vi "TCP Server 全双工.vi"() -> ()   [LabVIEW 2015]
uses:
  <vilib>/measure/NI_MABase.lvlib
panel:
  in  "stop 2":bool
  in  "stop":bool
  out "receive from client":dbl[](graph)
  in  "port":u16
  out "send to client":waveform(dbl)(graph)
  in  "signal type":T1(ring)
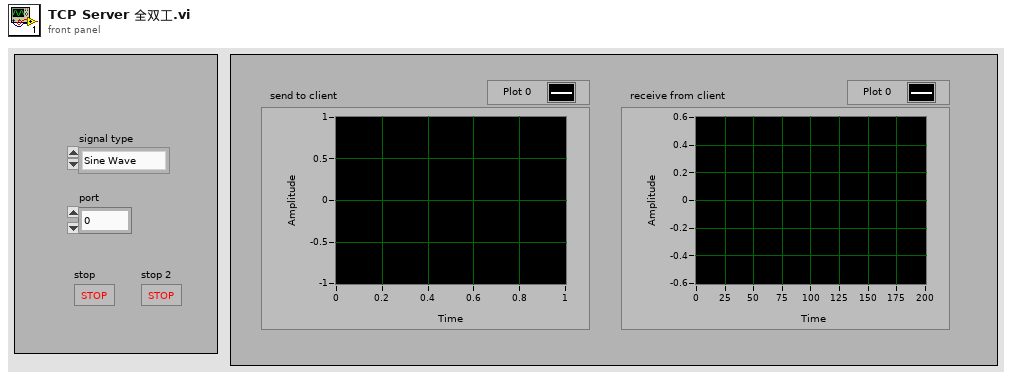
[diagram p1: front panel]
types:
  T1 = enum16{"Sine Wave", "Triangle Wave", "Square Wave", "Sawtooth Wave"}
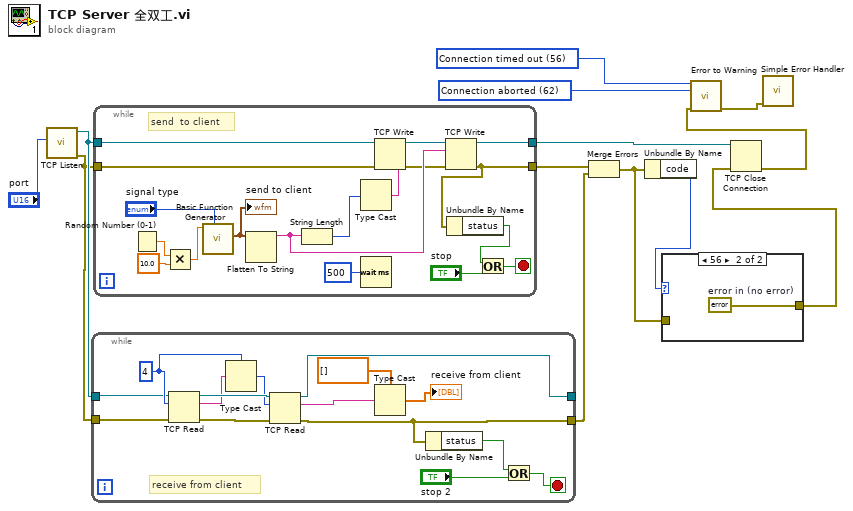
[diagram p0: block diagram]
diagram:
  w6 = 62 items=["No Error", "Argument Error", "Memory Full", "Out of Zone", "End of File", "File Already Open", "Generic File IO Error", "File Not Found", "File Permission Error", "Disk Full", "Duplicate Path", "Too Many Files Open", "Not Enabled", "Resource File Not Found", "Cannot Add Resource", "Resource Not Found", "Image Not Found", "Image Memory Error", "Pen Does Not Exist", "Config Bad Type", "Config Token Not Found", "Config Parse Error", "Config Memory Error", "Bad External Code Format", "Bad External Code Offset", "External Code Not Present", "Null Window", "Destroy Window Mixup", "Null Menu", "Print Aborted", "Bad Print Record", "Print Driver Error", "Windows Error During Print", "Memory Error During Print", "Print Dialog Error", "Generic Print Error", "Invalid Device Refnum", "Device Not Found", "Device Parameter Error", "Device Unit Error", "Can't Open Device", "Device Call Aborted", "Generic Error", "Cancelled By User", "Object ID Too Low", "Object ID Too High", "Object Not In Heap", "Unknown Heap", "Bad DefProc ID", "DefProc Not In Table", "Message Out Of Range", "Null Method", "Unknown Message", "Manager Call Not Supported", "Bad address", "Connection In progress", "Connection timed out", "Connection is already in progress", "Network attribute not supported", "Network error", "Address in use", "System out of memory", "Connection aborted", "Connection refused", "Connection is not connected", "Connection is already connected", "Connection closed", "Initialize error (interapplication manager)", "Bad occurrence", "Wait on unbound occurrence handler", "Occurrence queue overflow", "Bad path", "Semaphore not signaled", "Unrecognized type (interapplication manager)"] ("2nd Error to Convert")
  w7 = 56 items=["No Error", "Argument Error", "Memory Full", "Out of Zone", "End of File", "File Already Open", "Generic File IO Error", "File Not Found", "File Permission Error", "Disk Full", "Duplicate Path", "Too Many Files Open", "Not Enabled", "Resource File Not Found", "Cannot Add Resource", "Resource Not Found", "Image Not Found", "Image Memory Error", "Pen Does Not Exist", "Config Bad Type", "Config Token Not Found", "Config Parse Error", "Config Memory Error", "Bad External Code Format", "Bad External Code Offset", "External Code Not Present", "Null Window", "Destroy Window Mixup", "Null Menu", "Print Aborted", "Bad Print Record", "Print Driver Error", "Windows Error During Print", "Memory Error During Print", "Print Dialog Error", "Generic Print Error", "Invalid Device Refnum", "Device Not Found", "Device Parameter Error", "Device Unit Error", "Can't Open Device", "Device Call Aborted", "Generic Error", "Cancelled By User", "Object ID Too Low", "Object ID Too High", "Object Not In Heap", "Unknown Heap", "Bad DefProc ID", "DefProc Not In Table", "Message Out Of Range", "Null Method", "Unknown Message", "Manager Call Not Supported", "Bad address", "Connection In progress", "Connection timed out", "Connection is already in progress", "Network attribute not supported", "Network error", "Address in use", "System out of memory", "Connection aborted", "Connection refused", "Connection is not connected", "Connection is already connected", "Connection closed", "Initialize error (interapplication manager)", "Bad occurrence", "Wait on unbound occurrence handler", "Occurrence queue overflow", "Bad path", "Semaphore not signaled", "Unrecognized type (interapplication manager)"] ("1st Error to Convert")
  n1 = call <vilib>:"TCP Listen.vi"("port"="port") -> ("error out"=w5:errorcluster, "connection ID"=w10:refnum<k5>)  [unwired: 6 in, 3 out]
  n2 = while {
    tunnel: [w22] -> _
    tunnel: [w16] -> w12
    tunnel: w10 -> [w21]
    tunnel: w5 -> [w19]
    stop <- w20 stop-if-true
    w26 = 4
    # "receive from client"
    n3 = TCP Read(connection ID=w21, bytes to read=w26, error in (no error)=w19) -> (connection ID out=w28:refnum<k5>, data out=w25:string, error out=w27:errorcluster)  [unwired: 2 in]
    n4 = Type Cast(type=w26, x=w25) -> (*(type *) &x=w24:i32)
    n5 = TCP Read(connection ID=w28, bytes to read=w24, error in (no error)=w27) -> (connection ID out=w22:refnum<k5>, data out=w23:string, error out=w16:errorcluster)  [unwired: 2 in]
    n6 = Type Cast(type=dbl[] [], x=w23) -> (*(type *) &x=→"receive from client":dbl[])
    n7 = Unbundle By Name(w16) -> ("status"=w18:bool)
    n8 = Or(x=w18, y="stop 2") -> (x .or. y?=w20:bool)
  }
  n9 = while {
    tunnel: [w36] -> w11
    tunnel: w10 -> [w35]
    tunnel: w5 -> [w34]
    tunnel: [w32] -> w9
    stop <- w33 stop-if-true
    # "send  to client"
    n10 = Random Number (0-1)() -> (number: 0 to 1=w45:dbl)
    n11 = Multiply(x=w45, y=10.0) -> (x*y=w43:dbl)
    n12 = call <vilib>:"Basic Function Generator.vi"("signal type"="signal type", "frequency"=w43) -> ("signal out"=w41:waveform(dbl))  [unwired: 7 in, 2 out]
    "send to client" <- w41
    n13 = Flatten To String(anything=w41) -> (data string=w39:string)  [unwired: 3 in, 2 out]
    n14 = String Length(string=w39) -> (length=w42:i32)
    n15 = Type Cast(x=w42) -> (*(type *) &x=w40:string)  [unwired: 1 in]
    n16 = Wait (ms)(milliseconds to wait=u32 500) -> ()  [unwired: 1 out]
    n17 = TCP Write(connection ID=w35, data in=w40, error in (no error)=w34) -> (connection ID out=w38:refnum<k5>, error out=w37:errorcluster)  [unwired: 1 in, 1 out]
    n18 = TCP Write(connection ID=w38, data in=w39, error in (no error)=w37) -> (connection ID out=w36:refnum<k5>, error out=w32:errorcluster)  [unwired: 1 in, 1 out]
    n19 = Unbundle By Name(w32) -> ("status"=w31:bool)
    n20 = Or(x=w31, y="stop") -> (x .or. y?=w33:bool)
  }
  n21 = Merge Errors(w9, w12) -> (w3:errorcluster)
  n22 = Unbundle By Name(w3) -> ("code"=w2:i32)
  n23 = case shown="56" w2 {
    tunnel: w3 -> [w47 _]
    tunnel: [w47 w48] -> w1
    frame Default {
    }
    frame 56 {
      w48 = errorcluster {"status"=TRUE, "code"=0, "source"=""}  # error in (no error)
    }
  }
  n24 = TCP Close Connection(connection ID=w11, error in (no error)=w1) -> (error out=w4:errorcluster)  [unwired: 1 in, 1 out]
  n25 = call <vilib>:"Error to Warning.vi"("1st Error to Convert"=w7, "2nd Error to Convert"=w6, "error in"=w4) -> ("warning out"=w8:errorcluster)  [unwired: 12 in]
  n26 = call <vilib>:"Simple Error Handler.vi"("error in (no error)"=w8) -> ()  [unwired: 4 in, 5 out]
